vi "Swerve Wheel.vi"(4 "Inputs":dbl[](array[numeric])=[-0.0, -0.0, 0.0, 0.0, 0.0, 14.0, 19.623009453190406, 13.75], 5 "Wheel":T1(ring)=enum."Front Left") -> (0 "Speed":dbl, 1 "Spin Motor Power":dbl, 2 "PID Tracking":cluster{"Goal Wheel Position":dbl, dbl}(graph)={"Goal Wheel Position"=0.0, -90.17571233858979})   [LabVIEW 2014]
doc: "Used within Swerve Drive.vi.\nControls an individual wheel."
uses:
  Global Variables/Settings.vi
  Global Variables/Sensor Data (Edited).vi
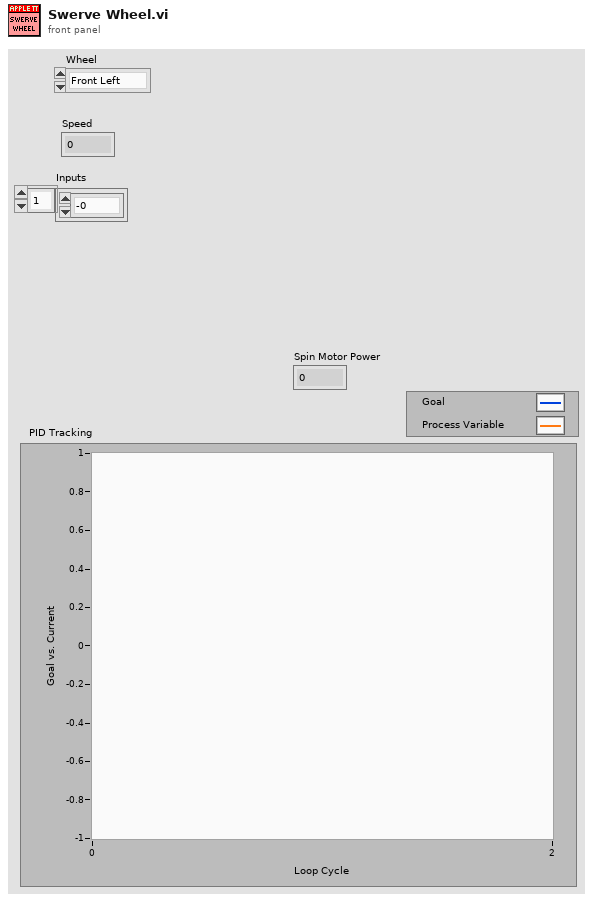
[diagram p1: front panel]
types:
  T1 = enum16{"Back Left", "Back Right", "Front Left", "Front Right"}
  T2 = enum16{"Z", "Y", "X", "Rot. Point X", "Rot. Point Y", "Width/2", "Max", "Length/2"}
  T3 = enum16{"Z Axis", "Y", "X", "Rot. Point X", "Rot. Point Y", "Width/2", "Max", "Length/2"}
  T4 = cluster{"proportional gain (Kc)":dbl, "integral time (Ti, min)":dbl, "derivative time (Td, min)":dbl, "Maximum Value":dbl, "Minimum Value":dbl, "epsilon":dbl}
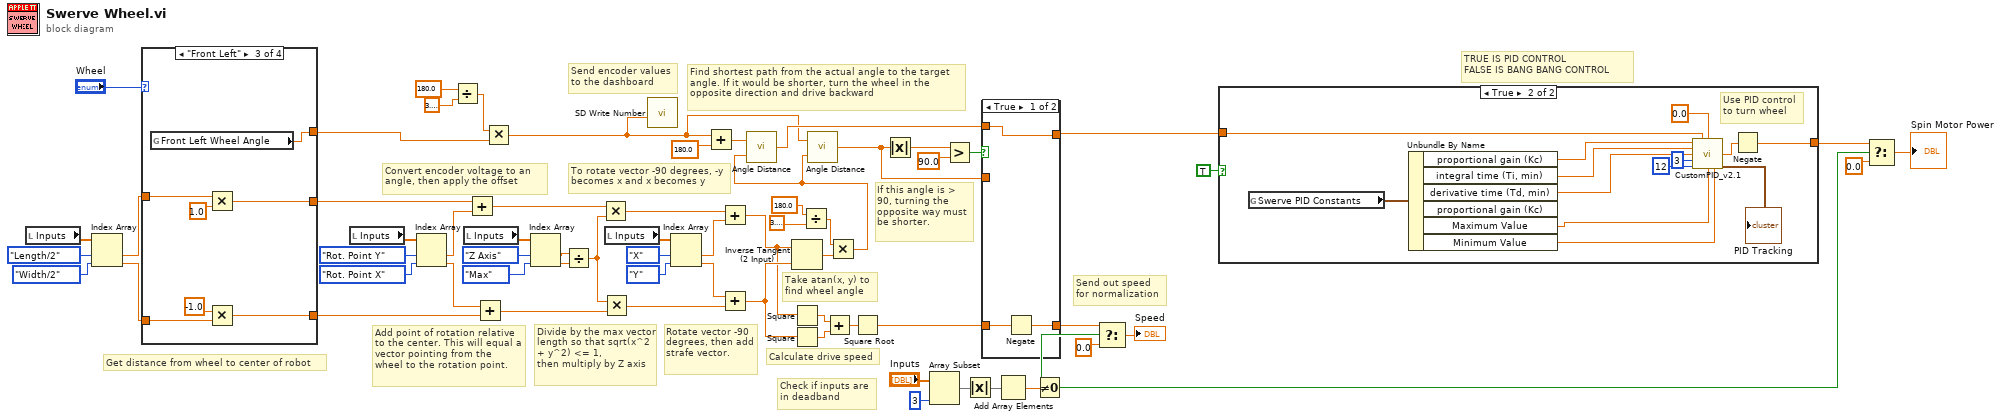
[diagram p0: block diagram]
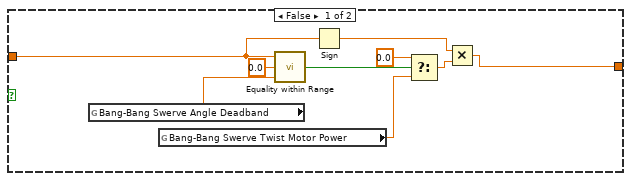
[diagram p2: hidden frame]
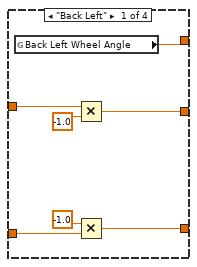
[diagram p4: hidden frame]
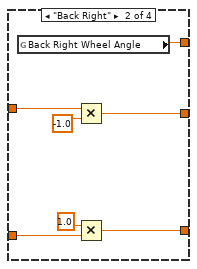
[diagram p5: hidden frame]
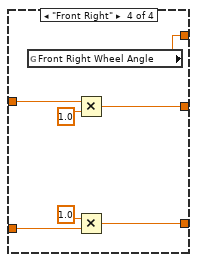
[diagram p6: hidden frame]
diagram:
  # "TRUE IS PID CONTROL\nFALSE IS BANG BANG CONTROL"
  # "Send encoder values \nto the dashboard"
  # "To rotate vector -90 degrees, -y becomes x and x becomes y"
  # "Divide by the max vector length so that sqrt(x^2 + y^2) <= 1,\nthen multiply by Z axis"
  # "Add point of rotation relative to the center. This will equal a vector pointing from the\nwheel to the rotation point."
  # "Send out speed\nfor normalization"
  # "Check if inputs are\nin deadband"
  # "Convert encoder voltage to an angle, then apply the offset"
  # "If this angle is > 90, turning the opposite way must be shorter."
  # "Find shortest path from the actual angle to the target angle. If it would be shorter, turn the wheel in the opposite direction and drive backward"
  # "Take atan(x, y) to find wheel angle"
  # "Calculate drive speed"
  # "Rotate vector -90 degrees, then add strafe vector."
  # "Get distance from wheel to center of robot"
  n1 = local read "Inputs"() -> (w17:dbl[])
  n2 = Index Array(array=w17, index #1=T2."Length/2", index #2=T2."Width/2") -> (element #1=w15:dbl, element #2=w14:dbl)
  n3 = case shown="\"Front Left\"" "Wheel" {
    tunnel: w15 -> [w71 w78 w85 w92]
    tunnel: w14 -> [w69 w76 w83 w90]
    tunnel: [w68 w75 w82 w89] -> w41
    tunnel: [w67 w74 w81 w88] -> w37
    tunnel: [w66 w73 w80 w87] -> w6
    frame "Back Left" {
      n4 = global read "Sensor Data (Edited).vi" "Back Left Wheel Angle"() -> (w66:dbl)
      n5 = Multiply(x=w71, y=-1.0) -> (x*y=w68:dbl)
      n6 = Multiply(x=-1.0 ("y"), y=w69) -> (x*y=w67:dbl)
    }
    frame "Back Right" {
      n7 = global read "Sensor Data (Edited).vi" "Back Right Wheel Angle"() -> (w73:dbl)
      n8 = Multiply(x=w78, y=-1.0) -> (x*y=w75:dbl)
      n9 = Multiply(x=1.0 ("y"), y=w76) -> (x*y=w74:dbl)
    }
    frame "Front Left" {
      n10 = global read "Sensor Data (Edited).vi" "Front Left Wheel Angle"() -> (w80:dbl)
      n11 = Multiply(x=w85, y=1.0) -> (x*y=w82:dbl)
      n12 = Multiply(x=-1.0 ("y"), y=w83) -> (x*y=w81:dbl)
    }
    frame "Front Right" {
      n13 = global read "Sensor Data (Edited).vi" "Front Right Wheel Angle"() -> (w87:dbl)
      n14 = Multiply(x=w92, y=1.0) -> (x*y=w89:dbl)
      n15 = Multiply(x=1.0 ("y"), y=w90) -> (x*y=w88:dbl)
    }
  }
  n16 = local read "Inputs"() -> (w39:dbl[])
  n17 = Index Array(array=w39, index #1=T2."Rot. Point Y", index #2=T2."Rot. Point X") -> (element #1=w35:dbl, element #2=w36:dbl)
  n18 = Divide(x=180.0, y=3.141592653589793) -> (x/y=w7:dbl)
  n19 = local read "Inputs"() -> (w33:dbl[])
  n20 = Add(x=w41, y=w35) -> (x+y=w12:dbl)
  n21 = Add(x=w36, y=w37) -> (x+y=w29:dbl)
  n22 = Multiply(x=w7, y=w6) -> (x*y=w4:dbl)
  n23 = Index Array(array=w33, index #1=T3."Z Axis", index #2=T2."Max") -> (element #1=w30:dbl, element #2=w31:dbl)
  n24 = Divide(x=w30, y=w31) -> (x/y=w28:dbl)
  n25 = Multiply(x=w12, y=w28) -> (x*y=w1:dbl)
  n26 = Multiply(x=w28, y=w29) -> (x*y=w23:dbl)
  n27 = local read "Inputs"() -> (w26:dbl[])
  n28 = call <vilib>:"SD Write Number.vi"("Numeric"=w4) -> ()  [unwired: 9 in, 2 out]
  n29 = Index Array(array=w26, index #1=T2."X", index #2=T2."Y") -> (element #1=w21:dbl, element #2=w22:dbl)
  n30 = Add(x=w4, y=180.0 ("f")) -> (x+y=w50:dbl)
  n31 = Add(x=w1, y=w21) -> (x+y=w19:dbl)
  n32 = Add(x=w22, y=w23) -> (x+y=w20:dbl)
  n33 = Inverse Tangent (2 Input)(1:w20, 2:w19) -> (0:w62:dbl)
  n34 = Square(x=w19) -> (x^2=w24:dbl)
  n35 = Square(x=w20) -> (x^2=w61:dbl)
  n36 = Divide(x=180.0 ("y"), y=3.141592653589793) -> (x/y=w59:dbl)
  n37 = Add(x=w24, y=w61) -> (x+y=w60:dbl)
  n38 = Multiply(x=w59, y=w62) -> (x*y=w13:dbl)
  n39 = call "Angle Distance.vi"("target angle"=w13, "current angle"=w50) -> ("distance"=w10:dbl)
  n40 = call "Angle Distance.vi"("target angle"=w13, "current angle"=w4) -> ("distance"=w53:dbl)
  n41 = Square Root(x=w60) -> (sqrt(x)=w52:dbl)
  n42 = Absolute Value(x=w53) -> (abs(x)=w54:dbl)
  n43 = Array Subset(array="Inputs", length=3) -> (w49:dbl[])  [unwired: 1 in]
  n44 = Greater?(x=w54, y=90.0) -> (0:w45:bool)
  n45 = Absolute Value(x=w49) -> (abs(x)=w42:dbl[])
  n46 = case shown="True" w45 {
    tunnel: w10 -> [w94 _]
    tunnel: w53 -> [_ w98]
    tunnel: [w95 w97] -> w48
    tunnel: w52 -> [w96 w97]
    tunnel: [w94 w98] -> w3
    frame True {
      n47 = Negate(x=w96) -> (-x=w95:dbl)
    }
    frame False {
    }
  }
  n48 = Add Array Elements(numeric array=w42) -> (sum=w63:dbl)
  n49 = Not Equal To 0?(x=w63) -> (x != 0?=w44:bool)
  n50 = Select(t=w48, s=w44, f=0.0) -> (s? t:f=→"Speed":dbl)
  n51 = case shown="True" TRUE {
    tunnel: [w103 w119] -> w43
    tunnel: w3 -> [w102 w117]
    frame False {
      n52 = global read "Settings.vi" "Bang-Bang Swerve Angle Deadband"() -> (w100:dbl)
      n53 = global read "Settings.vi" "Bang-Bang Swerve Twist Motor Power"() -> (w99:dbl)
      n54 = call "Equality within Range.vi"("Range"=w100, "Y"=0.0, "X"=w102) -> ("X = Y within Range?"=w106:bool)
      n55 = Sign(1:w102) -> (0:w101:dbl)
      n56 = Select(t=0.0, s=w106, f=w99) -> (s? t:f=w104:dbl)
      n57 = Multiply(x=w101, y=w104) -> (x*y=w103:dbl)
    }
    frame True {
      # "Use PID control\nto turn wheel"
      n58 = global read "Settings.vi" "Swerve PID Constants"() -> (w118:T4)
      n59 = Unbundle By Name(w118) -> ("proportional gain (Kc)"=w115:dbl, "integral time (Ti, min)"=w114:dbl, "derivative time (Td, min)"=w113:dbl, "Maximum Value"=w110:dbl, "Minimum Value"=w109:dbl)  [unwired: 1 out]
      n60 = call "CustomPID_v2.1.vi"("Kp"=w115, "Process Variable"=w117, "Goal"=0.0, "Ki"=w114, "Kd"=w113, "N-Diff"=3, "N-Int"=12, "Max Ouput"=w110, "Min Output"=w109) -> ("Command"=w120:dbl, "PID Tracking"=→"PID Tracking":cluster{"Goal Wheel Position":dbl, dbl})  [unwired: 4 in, 1 out]
      n61 = Negate(x=w120) -> (-x=w119:dbl)
    }
  }
  n62 = Select(t=w43, s=w44, f=0.0) -> (s? t:f=→"Spin Motor Power":dbl)
